vi "ADIS16448 Globals.vi"() -> ()   [LabVIEW 2019]
uses:
  Typedef/ADIS16448 Loop State.ctl
panel:
  out "IMU Detected":bool
  out "Calibrated?":bool
  out "Acquire Loop Count":i32
  out "CallOffsets":dbl[](array[numeric])
  out "Calibration Count":i32=-1
  out "Z-Mag":dbl
  out "Y-Mag":dbl
  out "X-Mag":dbl
  out "Baro Pressure":dbl
  out "Z-Accel":dbl
  out "Y-Accel":dbl
  out "X-Accel":dbl
  out "Temperature":dbl
  out "Z-Angle":dbl
  out "Y-Angle":dbl
  out "X-Angle":dbl
  in  "Loop State":T1
  # "DATA"
  # "DEBUG"
  # "STATUS"
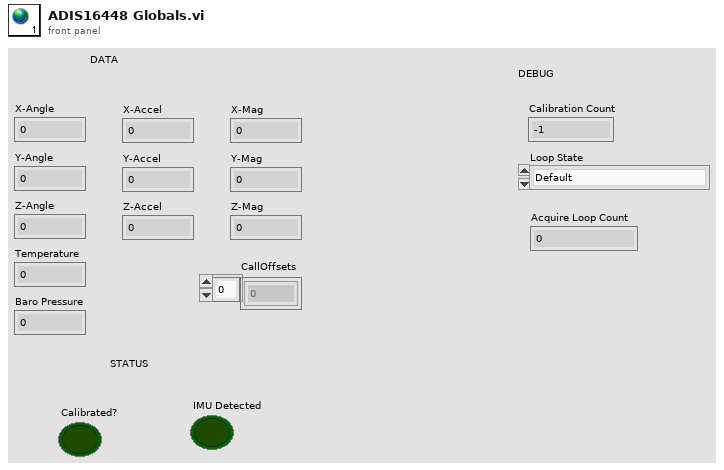
[diagram p1: front panel]
types:
  T1 = typedef "ADIS16448 Loop State.ctl" = enum16{"Default", "Error", "***Initialization***", "Reset", "Register DR Source", "Start SPI", "Write Config", "Init Auto SPI", "***Calibration***", "Calibrate", "Finish Cal", "***Operation***", "Run", "Process", "Run Cmds", "Run_Alt", "Run_Cmds_Alt", "Cal_Init_Alt", "Cal_Alt"}
diagram:
